vi "Set Loop Speed.vi"(8 "error in (no error)":errorcluster, 10 "Loop Speed":i32, 11 "Service in":refnum<class "Service.lvclass">) -> (0 "error out":errorcluster, 3 "Service out":refnum<class "Service.lvclass">)   [LabVIEW 2024, in "Ramses Framework.lvlib" / "Service.lvclass"]
uses:
  Service.lvclass
  Service.lvclass/Service.ctl
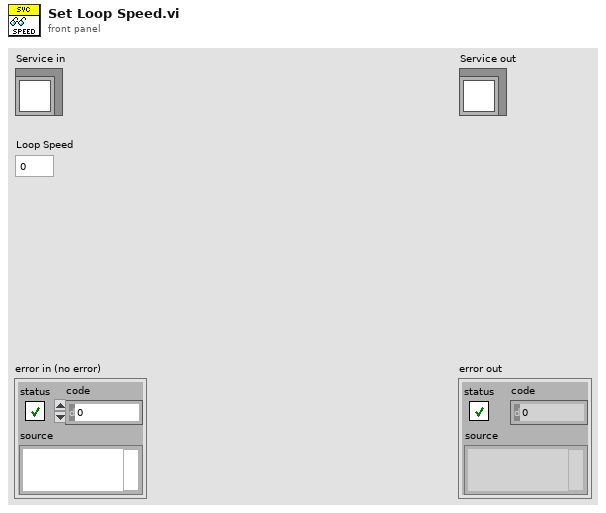
[diagram p1: front panel]
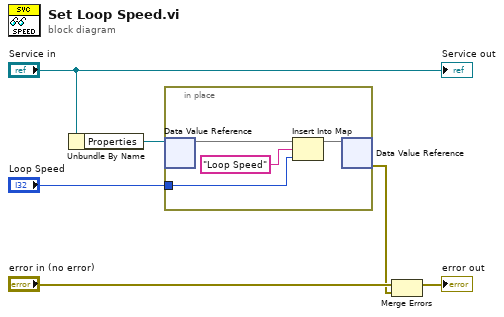
[diagram p0: block diagram]
diagram:
  n1 = Unbundle By Name("Service in") -> ("Properties"=w5:refnum<data-value>)
  n2 = in-place {
    in-place-border: "Loop Speed" -> [w7]
    n3 = in-place-dvr #1(w5) -> (w10:map{string, variant})  [unwired: 1 out]
    n4 = Insert Into Map(map in=w10, key="Loop Speed" ("Key"), value=w7) -> (map out=w9:map{string, variant})  [unwired: 2 out]
    n5 = in-place-dvr #1(w9) -> (w2:errorcluster)  [unwired: 1 out]
  }
  n6 = Merge Errors("error in (no error)", w2) -> (→"error out":errorcluster)
  "Service out" <- "Service in"
